vi "Add Log File.vi"(8 "error in (no error)":errorcluster, 10 "New Log":T1, 11 "Logs":T1[](array[typedef])) -> (0 "error out":errorcluster, 3 "Logs Out":T1[](array[typedef]))   [LabVIEW 2019]
uses:
  Controls/Log State.ctl
  Controls/Log.ctl
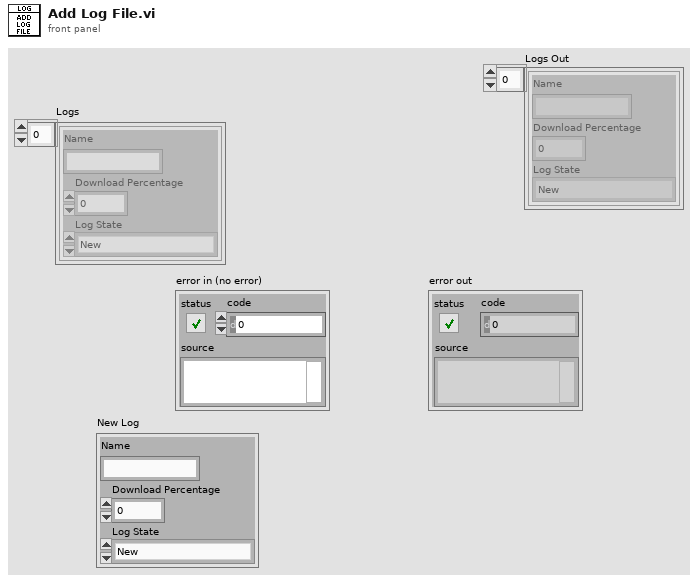
[diagram p1: front panel]
types:
  T1 = typedef "Log.ctl" = cluster{"Name":string, "Download Percentage":dbl, "Log State":T2}
  T2 = typedef "Log State.ctl" = enum16{"New", "Downloading", "Downloaded"}
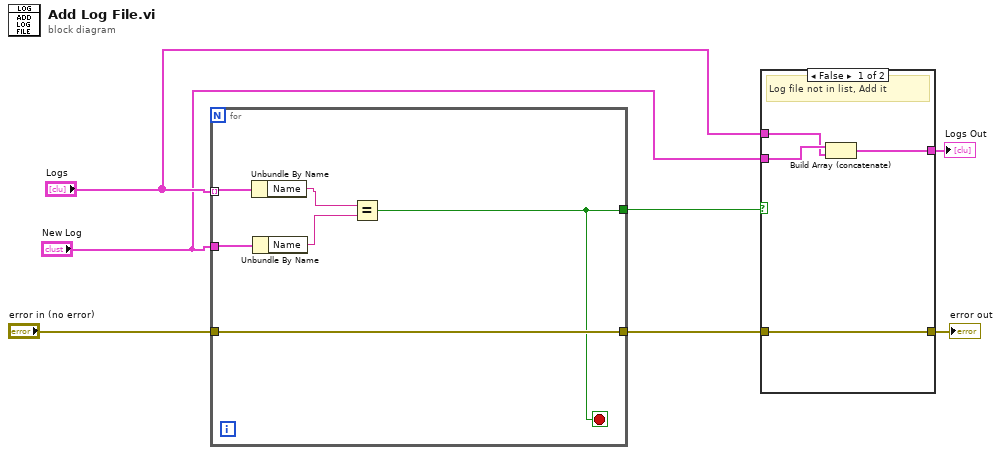
[diagram p0: block diagram]
diagram:
  n1 = for {
    tunnel: "Logs" -> [w12] mode=indexing
    tunnel: "New Log" -> [w11]
    tunnel: "error in (no error)" -> [w13]
    tunnel: [w13] -> w1
    tunnel: [w8] -> w6
    stop <- w8 stop-if-true
    n2 = Unbundle By Name(w12) -> ("Name"=w10:string)
    n3 = Unbundle By Name(w11) -> ("Name"=w9:string)
    n4 = Equal?(x=w10, y=w9) -> (x = y?=w8:bool)
  }
  n5 = case shown="False" w6 {
    tunnel: "Logs" -> [w16 w19]
    tunnel: "New Log" -> [w17 _]
    tunnel: [w15 w19] -> w3
    tunnel: [w14 w18] -> w2
    tunnel: w1 -> [w14 w18]
    frame False {
      # "Log file not in list, Add it"
      n6 = Build Array (concatenate)(w17, w16) -> (w15:T1[])
    }
    frame True {
      # "Log file in list so do nothing"
    }
  }
  "error out" <- w2
  "Logs Out" <- w3
